vi "Keithley 2002 Error Reader.vi"(2 "error in":T1, 3 "GPIB address":string="16") -> (0 "error out":T1, 1 "error message":string)   [LabVIEW 2020]
doc: "This VI is used to read back all the error messages stored in the error queue."
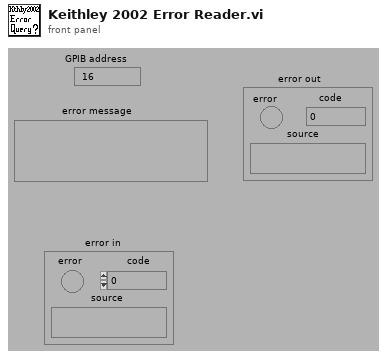
[diagram p1: front panel]
types:
  T1 = cluster{"error":bool, "code":i32, "source":string}
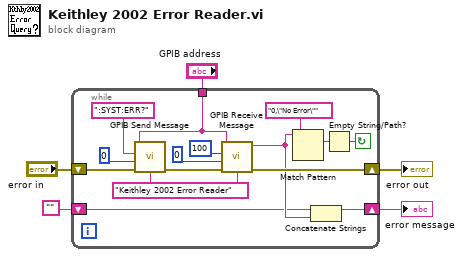
[diagram p0: block diagram]
diagram:
  n1 = while {
    tunnel: "GPIB address" -> [w11]
    shift-left: "error in" -> [w13]
    shift-right: [w12] -> w2
    shift-left: "" -> [w6]
    shift-right: [w7] -> w1
    stop <- w9 continue-if-true
    w14 = "Keithley 2002 Error Reader"
    n2 = call "GPIB Send Message.vi"("address string"=w11, "write buffer"=":SYST:ERR?", "source"=w14, "write mode (set END:0)"=0, "error in"=w13) -> ("error out"=w17:T1)  [unwired: 2 in, 2 out]
    n3 = call "GPIB Receive Message.vi"("address string"=w11, "byte count"=100, "source"=w14, "read mode"=0, "error in"=w17) -> ("read buffer"=w8:string, "error out"=w12:T1)  [unwired: 2 in, 1 out]
    n4 = Match Pattern(string=w8, regular expression="0,\"No Error\"") -> (match substring=w10:string)  [unwired: 1 in, 3 out]
    n5 = Concatenate Strings(w6, w8) -> (w7:string)
    n6 = Empty String/Path?(string/path=w10) -> (empty?=w9:bool)
  }
  "error out" <- w2
  "error message" <- w1
